vi "updateReplayControls.vi"(8 "error in (no error)":errorcluster, 10 "ReplayControls in":T1={"Slide"=0.0, "Enable"=FALSE, "FPS"=1000.0, "On"=FALSE, "Play"=FALSE, "CopyFile"=FALSE, "CopyFilePathRelativeToLogFolder"="teste1.txt", "ReadFromFile"=FALSE, "ReadPathRelativeToLogFolder"="teste1.txt", "FrameBufferSize"=10000.0, "Speed"=1.0, "FrameNumber"=0.0} {"Slide" scale=0.0..10.0}, 11 "Game in":refnum<class "Game.lvclass">) -> (0 "error out":errorcluster, 2 "ReplayControls out":T1={"Slide"=0.0, "Enable"=FALSE, "FPS"=1000.0, "On"=FALSE, "Play"=FALSE, "CopyFile"=FALSE, "CopyFilePathRelativeToLogFolder"="teste1.txt", "ReadFromFile"=FALSE, "ReadPathRelativeToLogFolder"="teste1.txt", "FrameBufferSize"=10000.0, "Speed"=1.0, "FrameNumber"=0.0} {"Slide" scale=0.0..10.0}, 3 "Game out":refnum<class "Game.lvclass">)   [LabVIEW 2020, in "Game.lvclass"]
uses:
  Game.lvclass
  ReplayControls.ctl
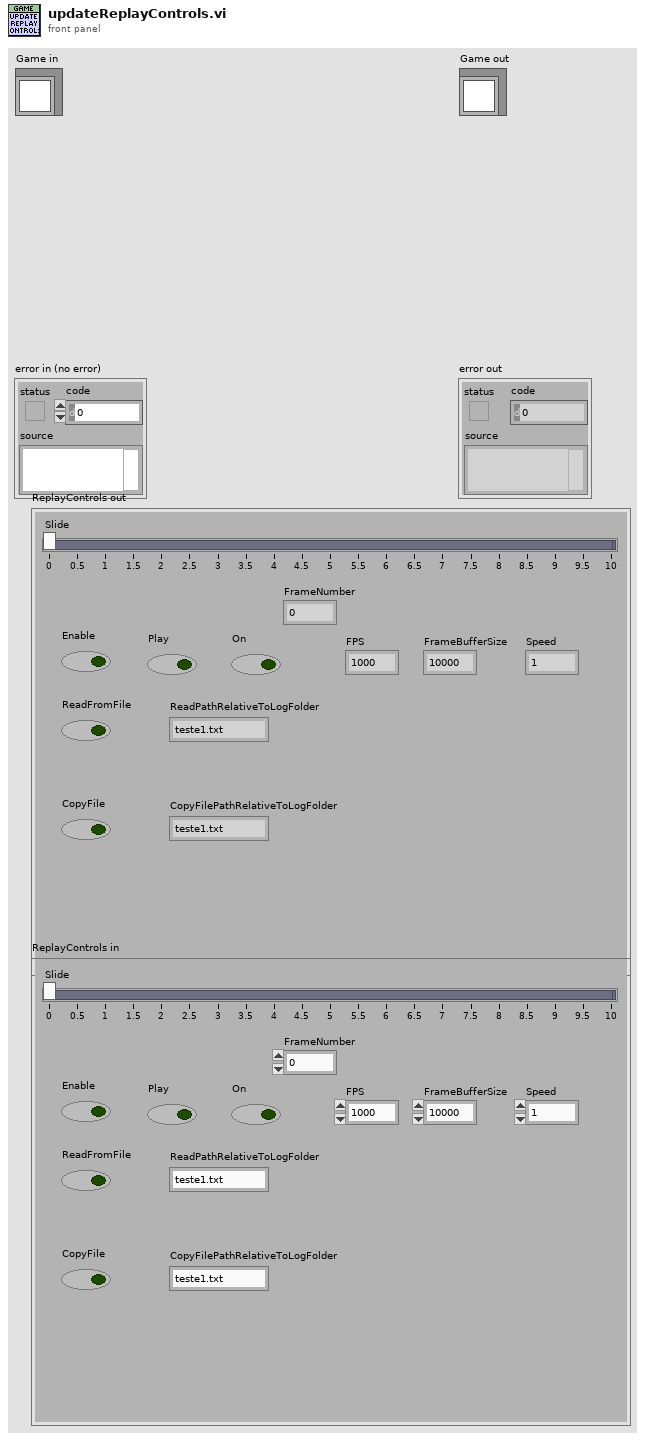
[diagram p1: front panel]
types:
  T1 = typedef "ReplayControls.ctl" = cluster{"Slide":dbl, "Enable":bool, "FPS":dbl, "On":bool, "Play":bool, "CopyFile":bool, "CopyFilePathRelativeToLogFolder":string, "ReadFromFile":bool, "ReadPathRelativeToLogFolder":string, "FrameBufferSize":dbl, "Speed":dbl, "FrameNumber":dbl}
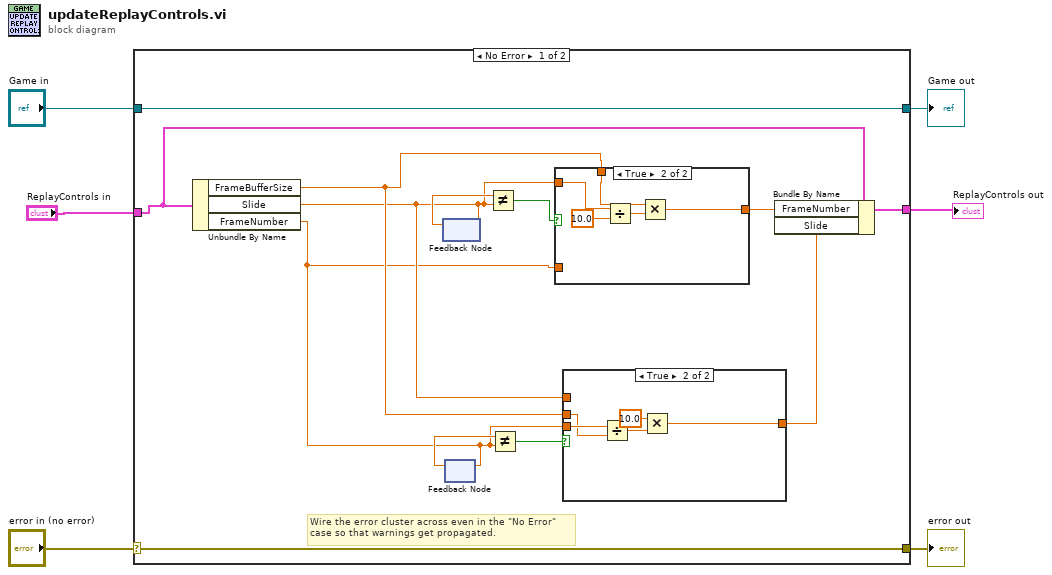
[diagram p0: block diagram]
diagram:
  n1 = case shown="No Error" "error in (no error)" {
    selector: "error in (no error)" -> [w18 w33]
    tunnel: [w18 w33] -> w5
    tunnel: [w19 w32] -> w3
    tunnel: "Game in" -> [w19 w32]
    tunnel: "ReplayControls in" -> [w17 _]
    tunnel: [w16 _] -> w1
    frame No Error {
      # "Wire the error cluster across even in the \"No Error\"\ncase so that warnings get propagated."
      n2 = Unbundle By Name(w17) -> ("FrameBufferSize"=w11:dbl, "Slide"=w8:dbl, "FrameNumber"=w7:dbl)
      n3 = feedback-in #1(w8) -> ()
      n4 = feedback #1() -> (w14:dbl)  [unwired: 1 in]
      n5 = feedback #2() -> (w10:dbl)  [unwired: 1 in]
      n6 = feedback-in #2(w7) -> ()
      n7 = Not Equal?(x=w14, y=w8) -> (x != y?=w15:bool)
      n8 = Not Equal?(x=w10, y=w7) -> (x != y?=w12:bool)
      n9 = case shown="True" w15 {
        tunnel: w7 -> [w26 _]
        tunnel: w8 -> [_ w31]
        tunnel: w11 -> [_ w28]
        tunnel: [w26 w27] -> w13
        frame False {
        }
        frame True {
          n10 = Divide(x=w31, y=10.0) -> (x/y=w29:dbl)
          n11 = Multiply(x=w28, y=w29) -> (x*y=w27:dbl)
        }
      }
      n12 = case shown="True" w12 {
        tunnel: w8 -> [w20 _]
        tunnel: w11 -> [_ w24]
        tunnel: w7 -> [_ w25]
        tunnel: [w20 w21] -> w9
        frame False {
        }
        frame True {
          n13 = Divide(x=w25, y=w24) -> (x/y=w23:dbl)
          n14 = Multiply(x=10.0, y=w23) -> (x*y=w21:dbl)
        }
      }
      n15 = Bundle By Name(cluster=w17, "FrameNumber"=w13, "Slide"=w9) -> (w16:T1)
    }
    frame Error {
    }
  }
  "error out" <- w5
  "Game out" <- w3
  "ReplayControls out" <- w1
